vi "Main.vi"() -> ()   [LabVIEW 2017]
doc: "This Continuous Measurement sample project is based on the Queued Message Handler template.\n\nThe Event Handling Loop generates messages based on user interface actions.\n\nThe Message Handling Loop processes messages generated by the Event Handling Loop, or by other messages. There are also Acquisition and Logging message handling loop subVIs, and a chart updating loop."
uses:
  Settings/Settings.ctl
  Acquisition/Hardware Configuration.ctl
  Acquisition/Signal Type.ctl
  Logging/Logging Configuration.ctl
  controls/UI Data.ctl
  controls/UI State.ctl
  support/Message Queue/Enqueue Message (Single).vi
  controls/ExitGlobal.vi
  support/Message Queue/Enqueue Message (Array).vi
  <vilib>/Utility/error.llb/Error Cluster From Error Code.vi
  <vilib>/ErrorRing/Error Ring.xnode
  Acquisition/Acquisition.lvlib
  Logging/Logging.lvlib
  Settings/Settings.lvlib
  support/User Event - Stop/User Event - Stop.lvlib
  support/Message Queue/Message Queue.lvlib
  Settings/Settings Dialog.vi
panel:
  out "Zero run":bool
  in  "Zero run?":bool
  out "Max writing time to a file [min]":dbl
  out "Test time zero run [s]":dbl
  out "Test time [min]":dbl
  in  "Start":bool
  in  "Stop":bool
  in  "Settings":bool
  out "Status":string
  in  "Exit":bool
  out "Log File Offsite Path":path
  out "Project code":string
  out "Offsite storage?":bool
  out "Log File Path":path
  out "Data":waveform(dbl)[](graph)
  # "Continuous Measurement Data Logger"
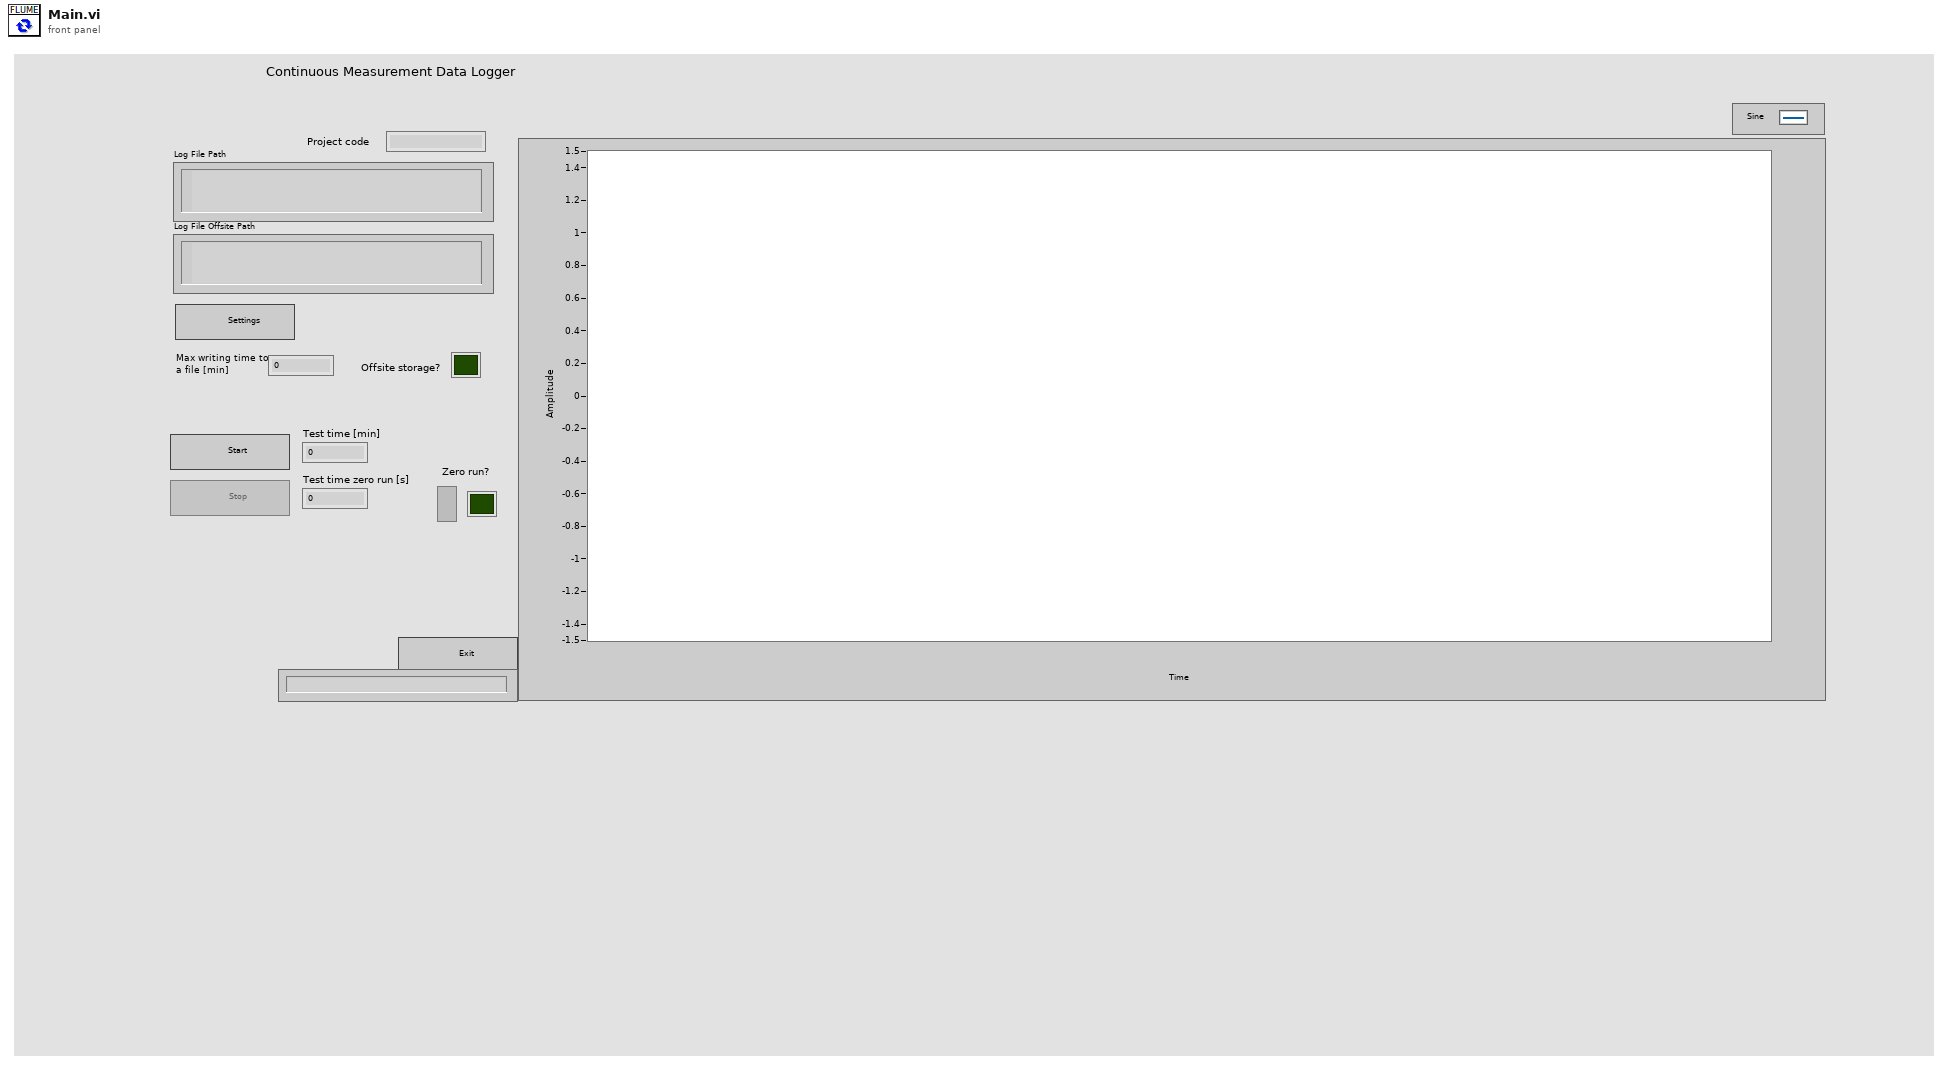
[diagram p1: front panel]
types:
  T1 = cluster{"Offsite storage?":bool, "Test time [s]":dbl, "Test time zero run [s] ":dbl, "Max writing time to a file [min]":dbl, "Zero run":bool}
  T2 = typedef "UI State.ctl" = enum16{"Idle", "Acquiring and Logging", "Waiting for Exit", "Waiting for Exit (Acq Stopped)", "Waiting for Exit (Log Stopped)", "Waiting for Stop", "Waiting for Stop (Acq Stopped)", "Waiting for Stop (Log Stopped)"}
  T3 = typedef "UI Data.ctl" = cluster{"Start Ref":refnum<vi>, "Stop Ref":refnum<vi>, "Settings Ref":refnum<vi>, "Exit Ref":refnum<vi>, "Status Ref":refnum<vi>, "Data Ref":refnum<vi>, "Zero run Ref":refnum<vi>}
  T4 = typedef "Settings.lvlib/Settings.ctl" = cluster{"Hardware Configuration":T5, "Logging Configuration":T7, "Timers":cluster{"Offsite storage?":bool, "Test time [s]":dbl, "Test time zero run [s] ":dbl, "Max writing time to a file [min]":dbl, "Zero run":bool}}
  T5 = typedef "Acquisition.lvlib/Hardware Configuration.ctl" = cluster{"HW Refnum <Replace Me>":string, "Signal Type <Replace Me>":T6}
  T6 = typedef "Acquisition.lvlib/Signal Type.ctl" = enum16{"Sine Wave", "Square with Noise"}
  T7 = typedef "Logging.lvlib/Logging Configuration.ctl" = cluster{"Log File Base Path":path, "TDMS File Reference":refnum<k34>, "Log File Offsite Path":path, "Project code":string, "Bin File Reference":refnum<file>}
  T8 = typedef "Message Queue.lvlib/All Message Queues.ctl" = cluster{"UI":refnum<queue>, "Acquisition":refnum<queue>, "Logging":refnum<queue>, "Bin Logging":refnum<queue>, "Time":refnum<queue>}
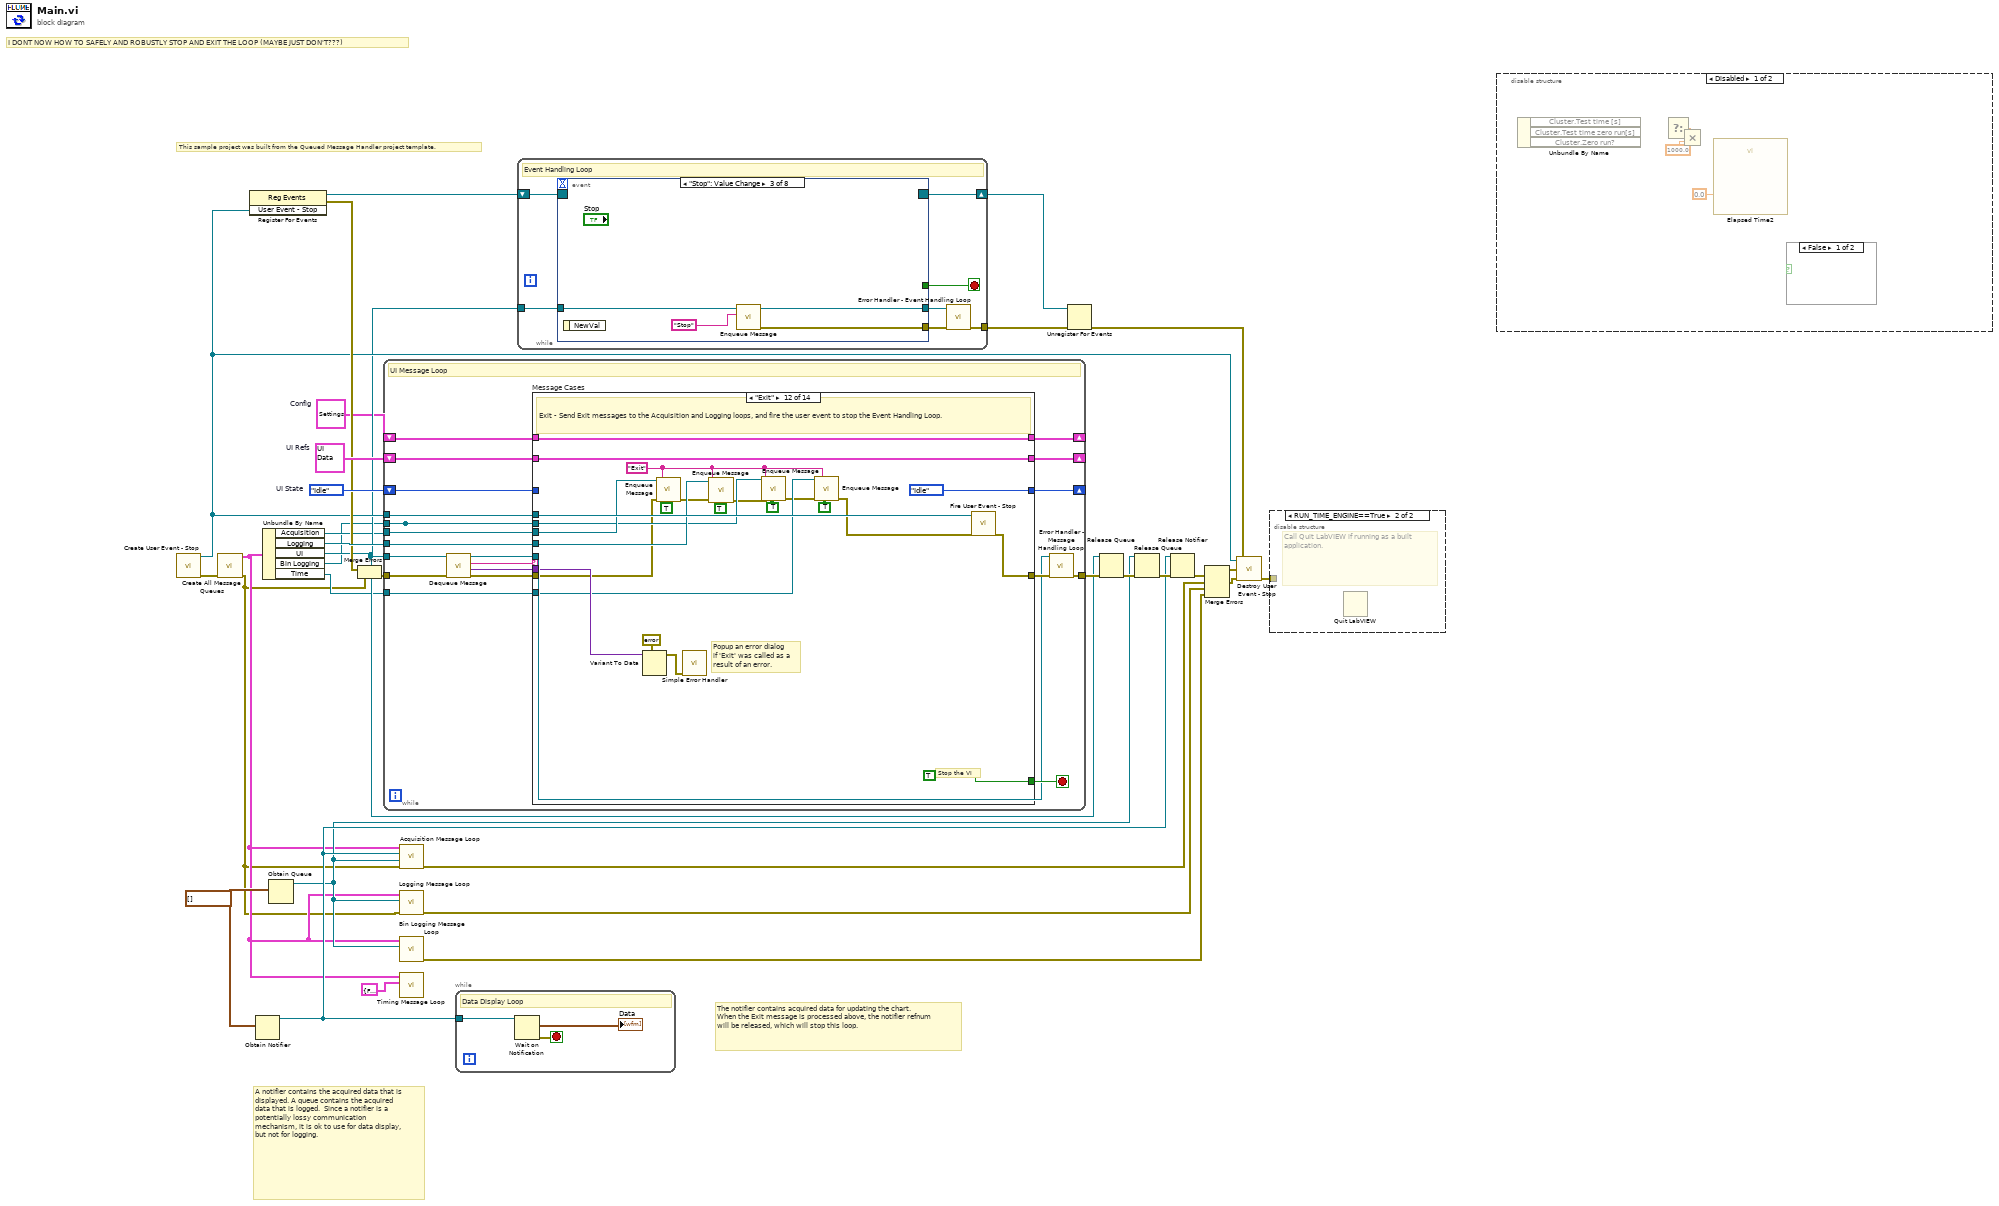
[diagram p0: block diagram]
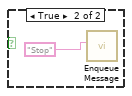
[diagram p2: hidden frame]
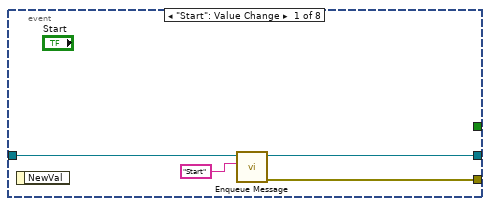
[diagram p5: hidden frame]
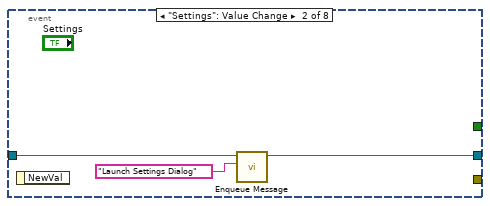
[diagram p6: hidden frame]
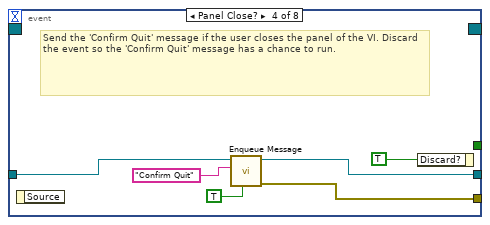
[diagram p7: hidden frame]
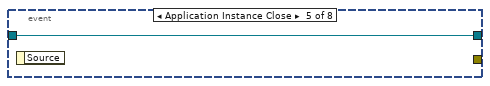
[diagram p8: hidden frame]
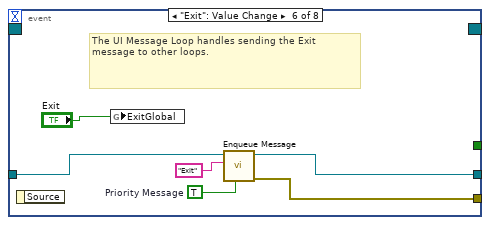
[diagram p9: hidden frame]
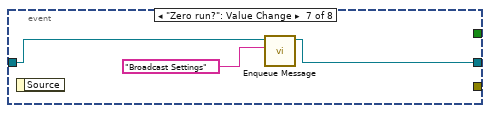
[diagram p10: hidden frame]
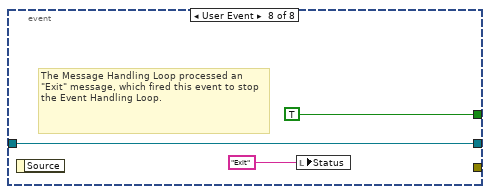
[diagram p11: hidden frame]
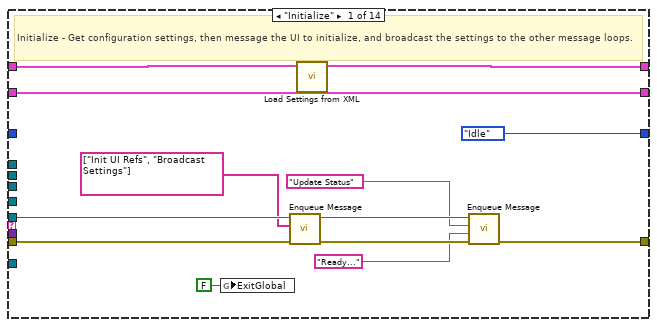
[diagram p12: hidden frame]
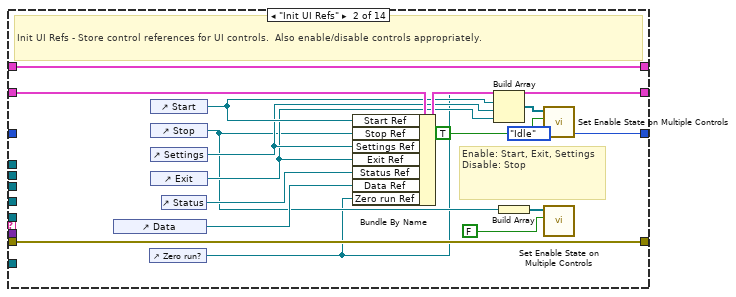
[diagram p13: hidden frame]
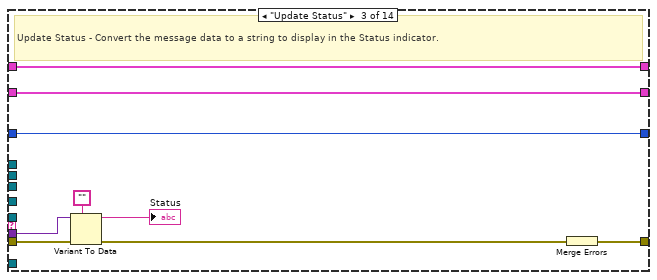
[diagram p14: hidden frame]
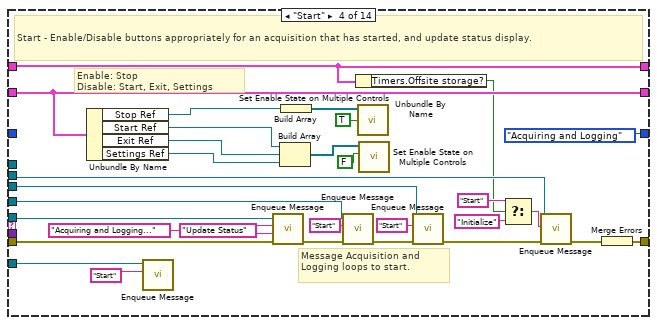
[diagram p15: hidden frame]
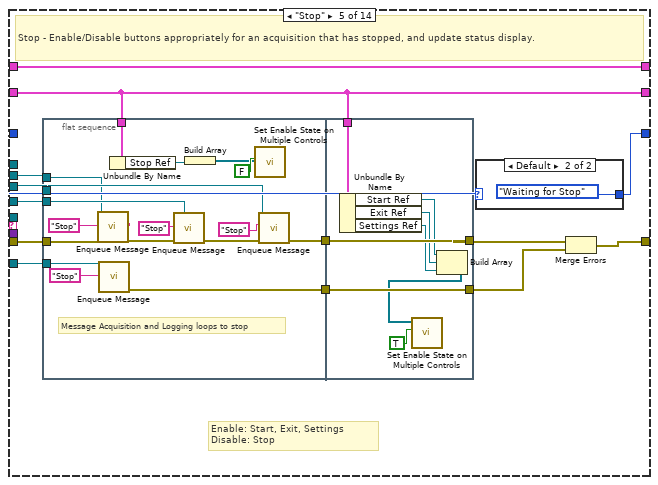
[diagram p16: hidden frame]
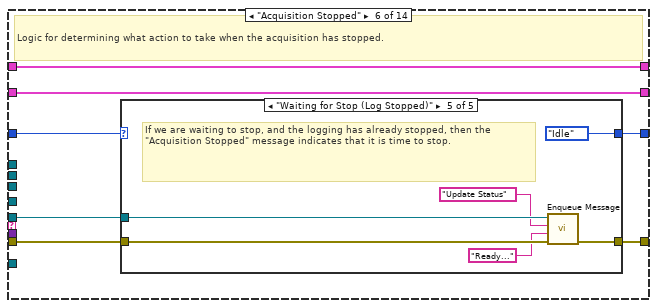
[diagram p18: hidden frame]
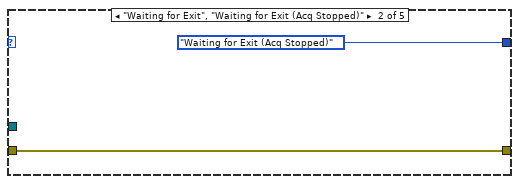
[diagram p20: hidden frame]
diagram:
  w25 = UI_State."Idle"  # UI State
  w10 = waveform(dbl)[] []
  w27 = T3 {"Start Ref"=refnum, "Stop Ref"=refnum, "Settings Ref"=refnum, "Exit Ref"=refnum, "Status Ref"=refnum, "Data Ref"=refnum, "Zero run Ref"=refnum}  # UI Refs
  w11 = T4 {"Hardware Configuration"={"HW Refnum <Replace Me>"="", "Signal Type <Replace Me>"=enum."Sine Wave"}, "Logging Configuration"={"Log File Base Path"=path "", "TDMS File Reference"=refnum, "Log File Offsite Path"=path "", "Project code"="", "Bin File Reference"=refnum}, "Timers"={"Offsite storage?"=FALSE, "Test time [s]"=10.0, "Test time zero run [s] "=180.0, "Max writing time to a file [min]"=30.0, "Zero run"=FALSE}}  # Config
  # "I DONT NOW HOW TO SAFELY AND ROBUSTLY STOP AND EXIT THE LOOP (MAYBE JUST DON'T???)"
  # "This sample project was built from the Queued Message Handler project template."
  # "A notifier contains the acquired data that is displayed. A queue contains the acquired data that is logged.  Since a notifier is a potentially lossy communication mechanism, it is ok to use for data display, but not for logging."
  # "The notifier contains acquired data for updating the chart. When the Exit message is processed above, the notifier refnum will be released, which will stop this loop."
  n1 = call "Create User Event - Stop.vi"() -> ("error out"=w29:errorcluster, "User Event - Stop"=w16:refnum<user-event>)  [unwired: 10 in]
  n2 = call "Create All Message Queues.vi"("error in (no error)"=w29) -> ("error out"=w1:errorcluster, "Message Queues out"=w5:T8)  [unwired: 9 in]
  n3 = register-events(w16) -> (reference out=w19:refnum<event-registration>, error out=w17:errorcluster)  [unwired: 2 in]
  n4 = Obtain Notifier(notification data type=w10) -> (notifier out=w12:refnum<notifier>)  [unwired: 3 in, 2 out]
  n5 = Unbundle By Name(w5) -> ("Acquisition"=w14:refnum<queue>, "Logging"=w26:refnum<queue>, "UI"=w15:refnum<queue>, "Bin Logging"=w8:refnum<queue>, "Time"=w4:refnum<queue>)
  n6 = Obtain Queue(element data type=w10) -> (queue out=w9:refnum<queue>)  [unwired: 4 in, 2 out]
  n7 = Merge Errors(w17, w1) -> (w18:errorcluster)
  n8 = while {
    tunnel: w15 -> [w38]
    tunnel: w16 -> [w50]
    shift-right: [w45] -> _
    shift-left: w11 -> [w34]
    shift-right: [w44] -> _
    shift-left: w27 -> [w32]
    tunnel: w14 -> [w43]
    tunnel: w26 -> [w37]
    shift-right: [w39] -> _
    shift-left: w25 -> [w40]
    tunnel: w18 -> [w49]
    tunnel: [w42] -> w31
    tunnel: w8 -> [w35]
    tunnel: [w35] -> _
    tunnel: w4 -> [w33]
    stop <- w51 stop-if-true
    # "UI Message Loop"
    n9 = call "Dequeue Message.vi"("error in (no error)"=w49, "Message Queue"=w38) -> ("error out"=w48:errorcluster, "Message Data"=w46:variant, "Message"=w47:string, "dup Message Queue"=w36:refnum<queue>)  [unwired: 6 in]
    n10 = case "Message Cases" shown="\"Exit\"" w47 {
      selector: w47 -> [_ _ _ _ _ _ _ _ _ _ _ _ _ w317]
      tunnel: w36 -> [w57 _ _ w101 _ w164 w189 _ w242 _ w264 _ _ _]
      tunnel: w48 -> [w56 w80 w88 w95 w133 w165 w190 w213 w244 w252 w263 w292 w315 _]
      tunnel: [w61 w80 w89 w103 w134 w162 w187 w211 w238 w255 w262 w308 w314 w316] -> w41
      tunnel: [_ _ _ _ _ _ _ _ _ _ _ TRUE _ _] -> w51
      tunnel: w46 -> [_ _ w87 _ _ _ _ _ _ w256 _ w301 _ _]
      tunnel: w50 -> [_ _ _ _ _ _ _ _ _ _ _ w309 _ _]
      tunnel: [w64 w67 w81 w94 w128 w161 w186 w215 w237 w251 w260 w299 w313 w320] -> w45
      tunnel: w34 -> [w53 w67 w81 w94 w128 w161 w186 w224 w245 w251 w260 w299 w313 w320]
      tunnel: w32 -> [w58 w79 w83 w118 w121 w167 w192 w234 w240 w259 w266 w307 w312 w319]
      tunnel: [w58 w76 w83 w118 w121 w167 w192 w234 w240 w259 w266 w307 w312 w319] -> w44
      tunnel: w43 -> [_ _ _ w102 w130 _ _ w233 _ _ _ w306 _ _]
      tunnel: w37 -> [_ _ _ w107 w132 _ _ w232 _ _ _ w305 _ _]
      tunnel: w40 -> [_ _ w82 _ w124 w166 w191 w231 w239 w254 w265 _ w311 w318]
      tunnel: [UI_State."Idle" ("UI State") UI_State."Idle" ("UI State") w82 UI_State."Acquiring and Logging" ("UI State") w129 w163 w188 w231 w239 w254 w261 UI_State."Idle" ("UI State") w311 w318] -> w39
      tunnel: w35 -> [_ _ _ w100 w127 _ _ w226 _ _ _ w298 _ _]
      tunnel: w33 -> [_ _ _ w98 w126 _ _ w223 _ _ _ w297 _ _]
      frame "Initialize" {
        # "Initialize - Get configuration settings, then message the UI to initialize, and broadcast the settings to the other message loops."
        n11 = global write "ExitGlobal.vi" "ExitGlobal"(FALSE ("ExitGlobal")) -> ()
        n12 = call-poly "Enqueue Message.vi"("error in (no error)"=w56, "Message Array"=string[] ["Init UI Refs", "Broadcast Settings"], "Message Queue"=w57) -> ("error out"=w63:errorcluster, "dup Message Queue"=w62:refnum<queue>)  [unwired: 7 in]
        n13 = call "Load Settings from XML.vi"("Settings in"=w53) -> ("Settings out"=w64:T4)  [unwired: 9 in, 1 out]
        n14 = call-poly "Enqueue Message.vi"("error in (no error)"=w63, "Message Data"="Ready..." ("Ready..."), "Message"="Update Status", "Message Queue"=w62) -> ("error out"=w61:errorcluster)  [unwired: 6 in, 1 out]
      }
      frame "Init UI Refs" {
        # "Enable: Start, Exit, Settings\nDisable: Stop"
        # "Init UI Refs - Store control references for UI controls.  Also enable/disable controls appropriately."
        n15 = control-ref of="Data"() -> (w77:refnum<vi>)
        n16 = control-ref of="Zero run?"() -> (w65:refnum<vi>)
        n17 = control-ref of="Start"() -> (w71:refnum<vi>)
        n18 = control-ref of="Stop"() -> (w66:refnum<vi>)
        n19 = control-ref of="Settings"() -> (w70:refnum<vi>)
        n20 = control-ref of="Exit"() -> (w69:refnum<vi>)
        n21 = control-ref of="Status"() -> (w78:refnum<vi>)
        n22 = Bundle By Name(cluster=w79, "Start Ref"=w71, "Stop Ref"=w66, "Settings Ref"=w70, "Exit Ref"=w69, "Status Ref"=w78, "Data Ref"=w77, "Zero run Ref"=w65) -> (w76:T3)
        n23 = Build Array(w65, w71, w70, w69) -> (w74:refnum<vi>[])
        n24 = Build Array(w66) -> (w73:refnum<vi>[])
        n25 = call "Set Enable State on Multiple Controls.vi"("Enable?"=TRUE, "Controls"=w74) -> ()  [unwired: 10 in]
        n26 = call "Set Enable State on Multiple Controls.vi"("Enable?"=FALSE, "Controls"=w73) -> ()  [unwired: 10 in]
      }
      frame "Update Status" {
        # "Update Status - Convert the message data to a string to display in the Status indicator."
        n27 = Variant To Data(error in=w88, type="", Variant=w87) -> (data=→"Status":string, error out=w85:errorcluster)
        n28 = Merge Errors(w85) -> (w89:errorcluster)
      }
      frame "Start" {
        # "Message Acquisition and Logging loops to start."
        # "Enable: Stop\nDisable: Start, Exit, Settings"
        # "Start - Enable/Disable buttons appropriately for an acquisition that has started, and update status display."
        n29 = Unbundle By Name(w118) -> ("Stop Ref"=w113:refnum<vi>, "Start Ref"=w112:refnum<vi>, "Exit Ref"=w111:refnum<vi>, "Settings Ref"=w110:refnum<vi>)
        n30 = call-poly "Enqueue Message.vi"("Message"="Start", "Message Queue"=w98) -> ()  [unwired: 8 in, 2 out]
        n31 = call-poly "Enqueue Message.vi"("error in (no error)"=w95, "Message Data"="Acquiring and Logging..." ("Acquiring and Logging..."), "Message"="Update Status", "Message Queue"=w101) -> ("error out"=w109:errorcluster)  [unwired: 6 in, 1 out]
        n32 = Build Array(w112, w111, w110) -> (w116:refnum<vi>[])
        n33 = Build Array(w113) -> (w115:refnum<vi>[])
        n34 = call-poly "Enqueue Message.vi"("error in (no error)"=w109, "Message"="Start", "Message Queue"=w107) -> ("error out"=w104:errorcluster)  [unwired: 7 in, 1 out]
        n35 = Unbundle By Name(w94) -> ("Timers.Offsite storage?"=w91:bool)
        n36 = call "Set Enable State on Multiple Controls.vi"("Enable?"=TRUE, "Controls"=w115) -> ()  [unwired: 10 in]
        n37 = call "Set Enable State on Multiple Controls.vi"("Enable?"=FALSE, "Controls"=w116) -> ()  [unwired: 10 in]
        n38 = call-poly "Enqueue Message.vi"("error in (no error)"=w104, "Message"="Start", "Message Queue"=w102) -> ("error out"=w97:errorcluster)  [unwired: 7 in, 1 out]
        n39 = Select(t="Start" ("Message"), s=w91, f="Initialize") -> (s? t:f=w90:string)
        n40 = call-poly "Enqueue Message.vi"("error in (no error)"=w97, "Message"=w90, "Message Queue"=w100) -> ("error out"=w96:errorcluster)  [unwired: 7 in, 1 out]
        n41 = Merge Errors(w96) -> (w103:errorcluster)
      }
      frame "Stop" {
        # "Enable: Start, Exit, Settings\nDisable: Stop"
        # "Stop - Enable/Disable buttons appropriately for an acquisition that has stopped, and update status display."
        n42 = flat-sequence {
          tunnel: w133 -> [w150]
          tunnel: w132 -> [w148]
          tunnel: w130 -> [w145]
          tunnel: w127 -> [w142]
          tunnel: w126 -> [w141]
          tunnel: [w146] -> w123
          tunnel: [w139] -> w122
          tunnel: w121 -> [w137]
          tunnel: [w157] -> w125
          tunnel: [w158] -> w131
          tunnel: w123 -> [w158]
          tunnel: w122 -> [w157]
          tunnel: w121 -> [w154]
          frame #0 {
            # "Message Acquisition and Logging loops to stop"
            n43 = call-poly "Enqueue Message.vi"("Message"="Stop", "Message Queue"=w142) -> ()  [unwired: 8 in, 2 out]
            n44 = call-poly "Enqueue Message.vi"("Message"="Stop", "Message Queue"=w141) -> ("error out"=w139:errorcluster)  [unwired: 8 in, 1 out]
            n45 = Unbundle By Name(w137) -> ("Stop Ref"=w136:refnum<vi>)
            n46 = call-poly "Enqueue Message.vi"("error in (no error)"=w150, "Message"="Stop", "Message Queue"=w148) -> ("error out"=w147:errorcluster)  [unwired: 7 in, 1 out]
            n47 = Build Array(w136) -> (w135:refnum<vi>[])
            n48 = call "Set Enable State on Multiple Controls.vi"("Enable?"=FALSE, "Controls"=w135) -> ()  [unwired: 10 in]
            n49 = call-poly "Enqueue Message.vi"("error in (no error)"=w147, "Message"="Stop", "Message Queue"=w145) -> ("error out"=w146:errorcluster)  [unwired: 7 in, 1 out]
          }
          frame #1 {
            n50 = Unbundle By Name(w154) -> ("Start Ref"=w153:refnum<vi>, "Exit Ref"=w152:refnum<vi>, "Settings Ref"=w151:refnum<vi>)
            n51 = Build Array(w153, w152, w151) -> (w156:refnum<vi>[])
            n52 = call "Set Enable State on Multiple Controls.vi"("Enable?"=TRUE, "Controls"=w156) -> ()  [unwired: 10 in]
          }
        }
        n53 = case shown="Default" w124 {
          selector: w124 -> [w159 _]
          tunnel: [w159 UI_State."Waiting for Stop" ("UI State")] -> w129
          frame "Waiting for Exit" {
          }
          frame Default {
          }
        }
        n54 = Merge Errors(w131, w125) -> (w134:errorcluster)
      }
      frame "Acquisition Stopped" {
        # "Logic for determining what action to take when the acquisition has stopped."
        n55 = case shown="\"Waiting for Stop (Log Stopped)\"" w166 {
          selector: w166 -> [w169 _ _ _ _]
          tunnel: w165 -> [w168 w171 w173 w179 w185]
          tunnel: w164 -> [_ _ _ w177 w182]
          tunnel: [w169 UI_State."Waiting for Exit (Acq Stopped)" ("UI State") UI_State."Waiting for Stop (Acq Stopped)" ("UI State") UI_State."Idle" ("UI State") UI_State."Idle" ("UI State")] -> w163
          tunnel: [w168 w171 w173 w178 w183] -> w162
          frame Default {
          }
          frame "Waiting for Exit", "Waiting for Exit (Acq Stopped)" {
          }
          frame "Waiting for Stop", "Waiting for Stop (Acq Stopped)" {
          }
          frame "Waiting for Exit (Log Stopped)" {
            # "If we are waiting to exit, and the logging has already stopped, then the \"Acquisition Stopped\" message indicates that it is time to exit."
            n56 = call-poly "Enqueue Message.vi"("Priority Message? (F)"=TRUE, "error in (no error)"=w179, "Message"="Exit", "Message Queue"=w177) -> ("error out"=w178:errorcluster)  [unwired: 6 in, 1 out]
          }
          frame "Waiting for Stop (Log Stopped)" {
            # "If we are waiting to stop, and the logging has already stopped, then the \"Acquisition Stopped\" message indicates that it is time to stop."
            n57 = call-poly "Enqueue Message.vi"("error in (no error)"=w185, "Message Data"="Ready..." ("Ready..."), "Message"="Update Status", "Message Queue"=w182) -> ("error out"=w183:errorcluster)  [unwired: 6 in, 1 out]
          }
        }
      }
      frame "Logging Stopped" {
        # "Logic for determining what action to take when the logging has stopped."
        n58 = case shown="Default" w191 {
          selector: w191 -> [w194 _ _ _ _]
          tunnel: w190 -> [w193 w196 w198 w204 w207]
          tunnel: w189 -> [_ _ _ w202 w206]
          tunnel: [w194 UI_State."Waiting for Exit (Log Stopped)" ("UI State") UI_State."Waiting for Stop (Log Stopped)" ("UI State") UI_State."Idle" ("UI State") UI_State."Idle" ("UI State")] -> w188
          tunnel: [w193 w196 w198 w203 w205] -> w187
          frame Default {
          }
          frame "Waiting for Exit", "Waiting for Exit (Log Stopped)" {
          }
          frame "Waiting for Stop", "Waiting for Stop (Log Stopped)" {
          }
          frame "Waiting for Exit (Acq Stopped)" {
            # "If we are waiting to exit, and the acquisition has already stopped, then the \"Logging Stopped\" message indicates that it is time to exit."
            n59 = call-poly "Enqueue Message.vi"("Priority Message? (F)"=TRUE, "error in (no error)"=w204, "Message"="Exit", "Message Queue"=w202) -> ("error out"=w203:errorcluster)  [unwired: 6 in, 1 out]
          }
          frame "Waiting for Stop (Acq Stopped)" {
            # "If we are waiting to stop, and the acquisition has already stopped, then the \"Logging Stopped\" message indicates that it is time to stop."
            n60 = call-poly "Enqueue Message.vi"("error in (no error)"=w207, "Message Data"="Ready..." ("Ready..."), "Message"="Update Status", "Message Queue"=w206) -> ("error out"=w205:errorcluster)  [unwired: 6 in, 1 out]
          }
        }
      }
      frame "Broadcast settings" {
        w222 = "Update Settings" ("Message")
        # "Broadcast settings - Send the 'Update Settings' message to the Logging and Acquisition message loops."
        n61 = Bundle By Name(cluster=w224, "Timers.Zero run"="Zero run?") -> (w215:T4)
        n62 = Unbundle By Name(w215) -> ("Hardware Configuration"=w235:T5, "Logging Configuration"=w216:T7, "Timers"=w221:T1)
        n63 = Unbundle By Name(w221) -> ("Max writing time to a file [min]"=→"Max writing time to a file [min]":dbl, "Offsite storage?"=→"Offsite storage?":bool, "Test time [s]"=→"Test time [min]":dbl, "Test time zero run [s]"=→"Test time zero run [s]":dbl)
        n64 = call-poly "Enqueue Message.vi"("error in (no error)"=w213, "Message Data"=w216, "Message"=w222, "Message Queue"=w226) -> ("error out"=w214:errorcluster)  [unwired: 6 in, 1 out]
        n65 = Unbundle By Name(w216) -> ("Log File Base Path"=→"Log File Path":path, "Log File Offsite Path"=→"Log File Offsite Path":path, "Project code"=→"Project code":string)
        n66 = Unbundle By Name(w215) -> ("Timers"=w219:T1)
        n67 = call-poly "Enqueue Message.vi"("error in (no error)"=w214, "Message Data"=w235, "Message"=w222, "Message Queue"=w233) -> ("error out"=w236:errorcluster)  [unwired: 6 in, 1 out]
        n68 = call-poly "Enqueue Message.vi"("error in (no error)"=w236, "Message Data"=w216, "Message"=w222, "Message Queue"=w232) -> ("error out"=w212:errorcluster)  [unwired: 6 in, 1 out]
        n69 = call-poly "Enqueue Message.vi"("error in (no error)"=w212, "Message Data"=w219, "Message"=w222, "Message Queue"=w223) -> ("error out"=w211:errorcluster)  [unwired: 6 in, 1 out]
        "Zero run" <- "Zero run?"
      }
      frame "Launch Settings Dialog" {
        # "Launch Settings Dialog - Launch the Settings Dialog when the user clicks the 'Settings' button."
        n70 = call-by-ref "?"("error in (no error)"=w244, "Settings in"=w245) -> ("error out"=w241:errorcluster, "Cancelled?"=w243:bool, "Settings out"=w237:T4)  [unwired: 8 in, 3 out]
        n71 = case shown="False" w243 {
          tunnel: w242 -> [w249 _]
          tunnel: w241 -> [w248 w250]
          tunnel: [w247 w250] -> w238
          frame False {
            n72 = call-poly "Enqueue Message.vi"("error in (no error)"=w248, "Message"="Broadcast Settings", "Message Queue"=w249) -> ("error out"=w247:errorcluster)  [unwired: 7 in, 1 out]
          }
          frame True {
          }
        }
      }
      frame "Error" {
        # "Error - Display an error dialog. This message is sent by the \"Error Handler\" VIs at the end of other loops in this application."
        n73 = Variant To Data(error in=w252, type=errorcluster {"status"=FALSE, "code"=0, "source"=""} ("error constant"), Variant=w256) -> (data=w253:errorcluster, error out=w257:errorcluster)
        n74 = call <vilib>:"Simple Error Handler.vi"("error in (no error)"=w253) -> ()  [unwired: 4 in, 5 out]
        n75 = Merge Errors(w257) -> (w255:errorcluster)
      }
      frame "Confirm Quit" {
        # "Confirm Quit - Message that can confirm whether or not the user wants to exit the application."
        n76 = case shown="\"Acquiring and Logging\"" w265 {
          tunnel: w264 -> [w272 w276]
          tunnel: w263 -> [w271 w275]
          tunnel: [w270 w274] -> w262
          tunnel: [UI_State."Idle" ("UI State") w273] -> w261
          frame Default {
            # "If 'Confirm Quit' comes in while the system is idle, there is no need for a confirmation message."
            n77 = call-poly "Enqueue Message.vi"("Priority Message? (F)"=TRUE, "error in (no error)"=w271, "Message"="Exit", "Message Queue"=w272) -> ("error out"=w270:errorcluster)  [unwired: 6 in, 1 out]
          }
          frame "Acquiring and Logging" {
            n78 = Two Button Dialog(message="Are you sure you want to quit while the acquisition is running?" ("Confirm Quit Message"), 1:"No" ("No"), 2:"Yes" ("Yes")) -> (T button?=w277:bool)
            n79 = case shown="True" w277 {
              tunnel: w276 -> [_ w286]
              tunnel: w275 -> [w282 w287]
              tunnel: [w282 w285] -> w274
              tunnel: [UI_State."Acquiring and Logging" ("UI State") UI_State."Waiting for Exit" ("UI State")] -> w273
              frame False {
                # "User did not want to quit."
              }
              frame True {
                n80 = call-poly "Enqueue Message.vi"("error in (no error)"=w287, "Message"="Stop", "Message Queue"=w286) -> ("error out"=w285:errorcluster)  [unwired: 7 in, 1 out]
              }
            }
          }
        }
      }
      frame "Exit" {
        w294 = "Exit" ("Message")
        # "Popup an error dialog if 'Exit' was called as a result of an error."
        # "Stop the VI"
        # "Exit - Send Exit messages to the Acquisition and Logging loops, and fire the user event to stop the Event Handling Loop."
        n81 = Variant To Data(type=errorcluster {"status"=FALSE, "code"=0, "source"=""} ("error constant"), Variant=w301) -> (data=w300:errorcluster)  [unwired: 1 in, 1 out]
        n82 = call-poly "Enqueue Message.vi"("Priority Message? (F)"=TRUE, "error in (no error)"=w292, "Message"=w294, "Message Queue"=w306) -> ("error out"=w291:errorcluster)  [unwired: 6 in, 1 out]
        n83 = call <vilib>:"Simple Error Handler.vi"("error in (no error)"=w300) -> ()  [unwired: 4 in, 5 out]
        n84 = call-poly "Enqueue Message.vi"("Priority Message? (F)"=TRUE, "error in (no error)"=w291, "Message"=w294, "Message Queue"=w305) -> ("error out"=w290:errorcluster)  [unwired: 6 in, 1 out]
        n85 = call-poly "Enqueue Message.vi"("Priority Message? (F)"=TRUE, "error in (no error)"=w290, "Message"=w294, "Message Queue"=w298) -> ("error out"=w289:errorcluster)  [unwired: 6 in, 1 out]
        n86 = call-poly "Enqueue Message.vi"("Priority Message? (F)"=TRUE, "error in (no error)"=w289, "Message"=w294, "Message Queue"=w297) -> ("error out"=w288:errorcluster)  [unwired: 6 in, 1 out]
        n87 = call "Fire User Event - Stop.vi"("error in (no error)"=w288, "User Event - Stop"=w309) -> ("error out"=w308:errorcluster)  [unwired: 9 in]
      }
      frame "---Copy This Frame---" {
        # "Duplicate this frame when creating new messages.  Change this comment in the duplicated frame to describe this message."
        n88 = Merge Errors(w315) -> (w314:errorcluster)
      }
      frame Default {
        # "'Default' case only runs if there is a message that isn't defined in any of the other cases.  Output a programming error."
        n89 = xnode "Error Ring"("parameter 0"=w317) -> ("error out"=w316:errorcluster)
      }
    }
    n90 = call "Error Handler - Message Handling Loop.vi"("error in (no error)"=w41, "Message Queue"=w36) -> ("dup error in"=w42:errorcluster)  [unwired: 8 in, 1 out]
  }
  n91 = call "Acquisition Message Loop.vi"("error in (no error)"=w1, "Data Queue"=w9, "Data Notifier"=w12, "Message Queues"=w5) -> ("error out"=w3:errorcluster)  [unwired: 7 in]
  n92 = call "Logging Message Loop.vi"("error in (no error)"=w1, "Data Queue"=w9, "Message Queues"=w5) -> ("error out"=w7:errorcluster)  [unwired: 8 in]
  n93 = call "Bin Logging Message Loop.vi"("Data Queue"=w9, "Message Queues"=w5) -> ("error out"=w2:errorcluster)  [unwired: 9 in]
  n94 = call "Timing Message Loop.vi"("Timers"=T1 {"Offsite storage?"=FALSE, "Test time [s]"=0.0, "Test time zero run [s] "=0.0, "Max writing time to a file [min]"=0.0, "Zero run"=FALSE}, "Message Queues"=w5) -> ()  [unwired: 9 in, 1 out]
  n95 = while "Data Display Loop" {
    tunnel: w12 -> [w330]
    stop <- w329 stop-if-true
    # "Data Display Loop"
    n96 = Wait on Notification(notifier=w330) -> (notification=→"Data":waveform(dbl)[], error out=w329:errorcluster)  [unwired: 3 in, 2 out]
  }
  n97 = while {
    tunnel: w15 -> [w336]
    tunnel: [w333] -> w30
    shift-right: [w335] -> w28
    shift-left: w19 -> [w337]
    stop <- w334 stop-if-true
    # "Event Handling Loop"
    n98 = event shown="[2] \"Stop\": Value Change" {
      selector: w337 -> [_ _ _ _ _ _ _ _]
      dyn-events: [_ _ _ _ _ _ _ _] -> w335
      timeout: _ -> [_ _ _ _ _ _ _ _]
      tunnel: [_ _ _ _ _ _ _ TRUE ("Discard?")] -> w334
      tunnel: w336 -> [w341 w343 w347 w352 w355 w358 w363 w365]
      tunnel: [w339 _ w346 w350 _ w361 _ _] -> w332
      tunnel: [w338 w342 w345 w351 w355 w357 w362 w365] -> w331
      event "Start": Value Change {
        n99 = event-data() -> ()  [unwired: 1 in, 1 out]
        n100 = call-poly "Enqueue Message.vi"("Message"="Start", "Message Queue"=w341) -> ("error out"=w339:errorcluster, "dup Message Queue"=w338:refnum<queue>)  [unwired: 8 in]
      }
      event "Settings": Value Change {
        n101 = event-data() -> ()  [unwired: 1 in, 1 out]
        n102 = call-poly "Enqueue Message.vi"("Message"="Launch Settings Dialog", "Message Queue"=w343) -> ("dup Message Queue"=w342:refnum<queue>)  [unwired: 8 in, 1 out]
      }
      event "Stop": Value Change {
        n103 = event-data() -> ()  [unwired: 1 in, 1 out]
        n104 = call-poly "Enqueue Message.vi"("Message"="Stop", "Message Queue"=w347) -> ("error out"=w346:errorcluster, "dup Message Queue"=w345:refnum<queue>)  [unwired: 8 in]
      }
      event Panel Close? {
        # "Send the 'Confirm Quit' message if the user closes the panel of the VI. Discard the event so the 'Confirm Quit' message has a chance to run."
        n105 = event-data() -> ()  [unwired: 1 in, 1 out]
        n106 = call-poly "Enqueue Message.vi"("Priority Message? (F)"=TRUE, "Message"="Confirm Quit", "Message Queue"=w352) -> ("error out"=w350:errorcluster, "dup Message Queue"=w351:refnum<queue>)  [unwired: 7 in]
        n107 = event-data("Discard?"=TRUE) -> ()  [unwired: 1 in, 1 out]
      }
      event Application Instance Close {
        n108 = event-data() -> ()  [unwired: 1 in, 1 out]
      }
      event "Exit": Value Change {
        w359 = TRUE  # Priority Message
        # "The UI Message Loop handles sending the Exit message to other loops."
        n109 = event-data() -> ()  [unwired: 1 in, 1 out]
        n110 = global write "ExitGlobal.vi" "ExitGlobal"("Exit") -> ()
        n111 = call-poly "Enqueue Message.vi"("Priority Message? (F)"=w359, "Message"="Exit", "Message Queue"=w358) -> ("error out"=w361:errorcluster, "dup Message Queue"=w357:refnum<queue>)  [unwired: 7 in]
      }
      event "Zero run?": Value Change {
        n112 = event-data() -> ()  [unwired: 1 in, 1 out]
        n113 = call-poly "Enqueue Message.vi"("Message"="Broadcast Settings", "Message Queue"=w363) -> ("dup Message Queue"=w362:refnum<queue>)  [unwired: 8 in, 1 out]
      }
      event User Event {
        # "The Message Handling Loop processed an \"Exit\" message, which fired this event to stop the Event Handling Loop."
        n114 = event-data() -> ()  [unwired: 1 in, 1 out]
        n115 = local write "Status"("Exit" ("Exit String")) -> ()
      }
    }
    n116 = call "Error Handler - Event Handling Loop.vi"("error in (no error)"=w332, "Message Queue"=w331) -> ("dup error in"=w333:errorcluster)  [unwired: 8 in, 1 out]
  }
  n117 = Unregister For Events(event registration refnum=w28, error in=w30) -> (error out=w13:errorcluster)
  n118 = Release Queue(queue=w15, error in (no error)=w31) -> (error out=w22:errorcluster)  [unwired: 1 in, 2 out]
  n119 = Release Queue(queue=w9, error in (no error)=w22) -> (error out=w21:errorcluster)  [unwired: 1 in, 2 out]
  n120 = Release Notifier(notifier=w12, error in (no error)=w21) -> (error out=w20:errorcluster)  [unwired: 1 in, 2 out]
  n121 = Merge Errors(w13, w20, w3, w7, w2) -> (w24:errorcluster)
  n122 = call "Destroy User Event - Stop.vi"("error in (no error)"=w24, "User Event - Stop"=w16) -> ("error out"=w23:errorcluster)  [unwired: 9 in]
  n123 = disable-structure shown="RUN_TIME_ENGINE==True" {
    disable-tunnel: w23 -> [_ _]
    frame condition #0 (active) {
    }
    frame condition #1 {
      # "Call Quit LabVIEW if running as a built application."
      n124 = Quit LabVIEW() -> ()  [unwired: 1 in]
    }
  }
  n125 = disable-structure shown="Disabled" {
    frame Disabled {
      n126 = Unbundle By Name() -> ()  [unwired: 1 in, 3 out]
      n127 = Select() -> (s? t:f=w370:dbl)  [unwired: 3 in]
      n128 = Multiply(x=w370, y=1000.0) -> ()  [unwired: 1 out]
      n129 = call "Elapsed Time2"("Set Start Time (s)"=0.0) -> ()  [unwired: 11 in, 8 out]
      n130 = case shown="False" {
        selector: _ -> [_ _]
        frame False {
        }
        frame True {
          n131 = call-poly "Enqueue Message.vi"("Message"="Stop") -> ()  [unwired: 9 in, 2 out]
        }
      }
    }
    frame Enabled {
    }
  }
